vi "FTW-Connector-Ask.vi"(0 "FTW Actor Connector":refnum<class "FTW-Actor-Connector.lvclass">, 5 "Request Header":string, 7 "Request Body":string, 9 "Timeout":i32=100 format="%dmsec", 11 "error in":errorcluster) -> (4 "FTW Actor Connector out":refnum<class "FTW-Actor-Connector.lvclass">, 6 "Response Body":string, 8 "Roundtrip Time":dbl format="%.4psec", 15 "error out":errorcluster)   [LabVIEW 2014, in "FTW-Actor-Connector.lvclass"]
uses:
  FTW-Actor-Connector.lvclass
  FTW-Actor-Connector.lvclass/FTW-Actor-Connector.ctl
panel:
  # "Inputs"
  # "Outputs"
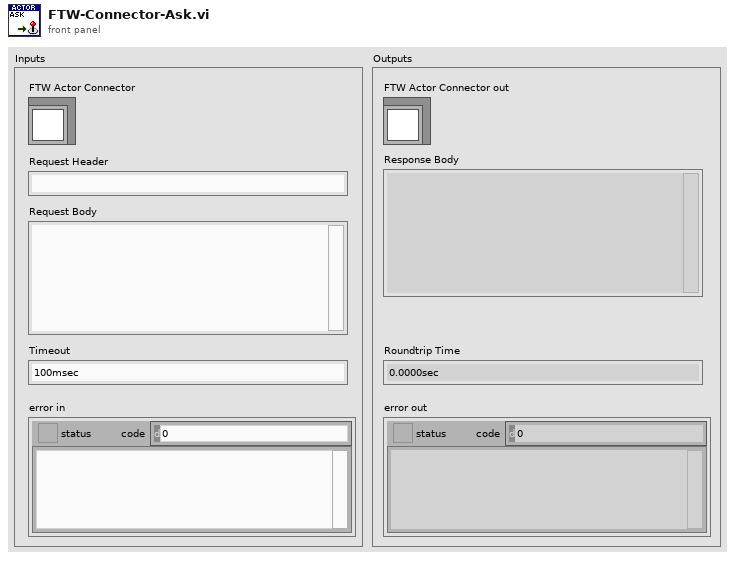
[diagram p1: front panel]
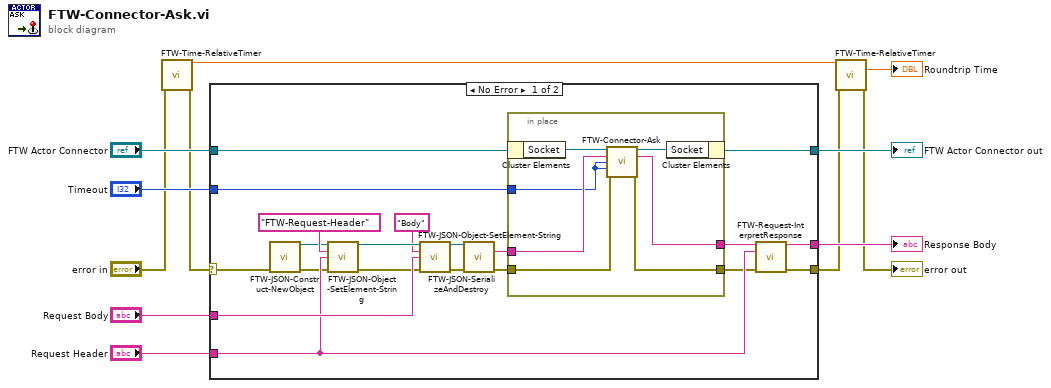
[diagram p0: block diagram]
diagram:
  n1 = call "FTW-Time-RelativeTimer.vi"("error in"="error in") -> ("Current Timer Value"=w6:dbl, "error out"=w4:errorcluster)  [unwired: 12 in, 1 out]
  n2 = case shown="No Error" w4 {
    selector: w4 -> [w13 w41]
    tunnel: "FTW Actor Connector" -> [w32 w40]
    tunnel: [w31 w40] -> w11
    tunnel: "Request Header" -> [w20 _]
    tunnel: "Request Body" -> [w29 _]
    tunnel: "Timeout" -> [w30 _]
    tunnel: [w17 _] -> w7
    tunnel: [w18 w41] -> w1
    frame No Error {
      n3 = call "FTW-JSON-Construct-NewObject.vi"("error in"=w13) -> ("JSON Object"=w15:refnum<data-value>, "error out"=w14:errorcluster)  [unwired: 13 in]
      n4 = call "FTW-JSON-Object-SetElement-String.vi"("JSON Object"=w15, "Key"="FTW-Request-Header", "Value"=w20, "error in"=w14) -> ("JSON Object out"=w27:refnum<data-value>, "error out"=w25:errorcluster)  [unwired: 10 in]
      n5 = call "FTW-JSON-Object-SetElement-String.vi"("JSON Object"=w27, "Key"="Body", "Value"=w29, "error in"=w25) -> ("JSON Object out"=w26:refnum<data-value>, "error out"=w24:errorcluster)  [unwired: 10 in]
      n6 = call "FTW-JSON-SerializeAndDestroy.vi"("JSON Object"=w26, "error in"=w24) -> ("JSON String (UTF-8)"=w28:string, "error out"=w16:errorcluster)  [unwired: 12 in]
      n7 = in-place {
        in-place-border: w16 -> [w35]
        in-place-border: [w39] -> w19
        in-place-border: w28 -> [w34]
        in-place-border: w30 -> [w33]
        in-place-border: [w36] -> w21
        n8 = in-place-cluster #1(w32) -> ("Socket"=w38:refnum<data-value>)
        n9 = call "FTW-Connector-Ask.vi"("FTW Actor Connector"=w38, "Request"=w34, "Receive Timeout"=w33, "Send Timeout"=w33, "error in"=w35) -> ("FTW Actor Connector out"=w37:refnum<data-value>, "Response"=w36:string, "error out"=w39:errorcluster)  [unwired: 7 in, 1 out]
        n10 = in-place-cluster #1("Socket"=w37) -> (w31:refnum<class "FTW-Actor-Connector.lvclass">)
      }
      n11 = call "FTW-Request-InterpretResponse.vi"("Raw Request"=w21, "Request Header"=w20, "error in"=w19) -> ("JSON Response"=w17:string, "error out"=w18:errorcluster)  [unwired: 11 in]
    }
    frame Error {
    }
  }
  "FTW Actor Connector out" <- w11
  "Response Body" <- w7
  n12 = call "FTW-Time-RelativeTimer.vi"("Previous Timer Value"=w6, "error in"=w1) -> ("Elapsed Time"=→"Roundtrip Time":dbl, "error out"=→"error out":errorcluster)  [unwired: 11 in, 1 out]
